vi "LEDs Streaming 2945 2955.vi"(0 "rx.parameters":T4={"rx.trigger select"=enum."Software", "rx.trigger enable"=FALSE, "rx.trigger sync enable"=FALSE, "rx.stream enable"=[FALSE, FALSE, FALSE, FALSE], "rx.software trigger"=FALSE, "rx.reset"=FALSE, "rx.abort"=FALSE, "rx.samples to acquire"=0, "rx.data sink"=enum."SFP Port 0", "rx.ddc parameters"=[{"output sample rate"=0.0, "delay"=0.0, "frequency shift"=0.0, "impairments"={"inline gain I"=0.0, "inline gain Q"=0.0, "cross gain I"=0.0, "cross gain Q"=0.0, "pre-gain offset I"=0.0, "pre-gain offset Q"=0.0, "post-gain offset I"=0.0, "post-gain offset Q"=0.0}, "phase"=0.0}, {"output sample rate"=0.0, "delay"=0.0, "frequency shift"=0.0, "impairments"={"inline gain I"=0.0, "inline gain Q"=0.0, "cross gain I"=0.0, "cross gain Q"=0.0, "pre-gain offset I"=0.0, "pre-gain offset Q"=0.0, "post-gain offset I"=0.0, "post-gain offset Q"=0.0}, "phase"=0.0}, {"output sample rate"=0.0, "delay"=0.0, "frequency shift"=0.0, "impairments"={"inline gain I"=0.0, "inline gain Q"=0.0, "cross gain I"=0.0, "cross gain Q"=0.0, "pre-gain offset I"=0.0, "pre-gain offset Q"=0.0, "post-gain offset I"=0.0, "post-gain offset Q"=0.0}, "phase"=0.0}, {"output sample rate"=0.0, "delay"=0.0, "frequency shift"=0.0, "impairments"={"inline gain I"=0.0, "inline gain Q"=0.0, "cross gain I"=0.0, "cross gain Q"=0.0, "pre-gain offset I"=0.0, "pre-gain offset Q"=0.0, "post-gain offset I"=0.0, "post-gain offset Q"=0.0}, "phase"=0.0}]} {"rx.ddc parameters"."frequency shift" format="%#.48g"}, 1 "rx.leds":T3, 5 "rx.status":T2={"rx.state"=enum."Idle", "rx.samples processed"=0, "rx.number of fifo overflows"=0, "rx.number of iq data overflows"=[0, 0, 0, 0], "rx.dsp reset done"=FALSE}) -> ()   [LabVIEW 2016]
uses:
  Stream Control State.ctl
  <vilib>/eio/EIONode/EIONode.xnode
  <vilib>/rvi/eio/common/nirviEmuTemplateMethod_errors.vi
  <instrlib>/_niInstr/Basic Elements/v1/FPGA/niInstr Basic Elements v1 FPGA.lvlib
  <instrlib>/_niInstr/Basic Elements/v1/FPGA/Private/Count Down U32.vi
  <instrlib>/_niInstr/DSP/v1/Shared/Public/IQ Impairments.ctl
  <instrlib>/_niInstr/DSP/v1/Shared/niInstr DSP v1 Shared.lvlib
  HOST/2954/SubVIs/Start Trigger.ctl
  DDC Parameters.ctl
  Rx Parameters.ctl
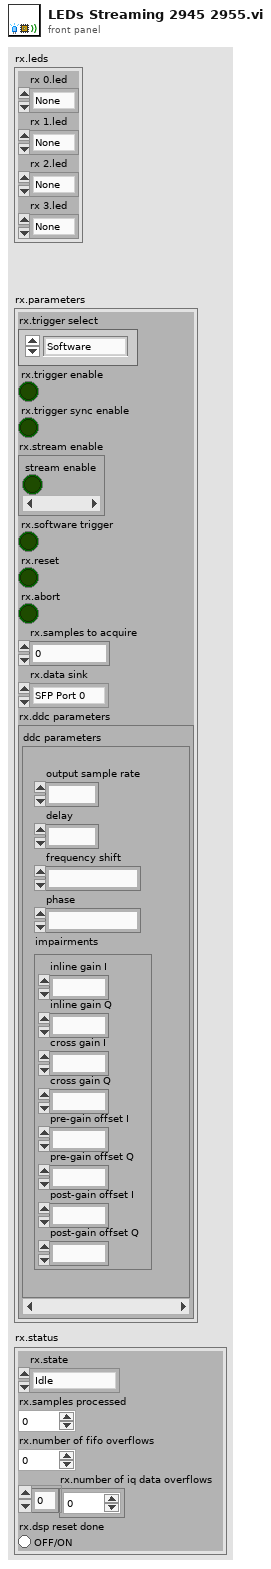
[diagram p1: front panel]
types:
  T1 = typedef "Stream Control State.ctl" = enum16{"Idle", "Active"}
  T2 = cluster{"rx.state":T1, "rx.samples processed":u32, "rx.number of fifo overflows":u32, "rx.number of iq data overflows":u64[], "rx.dsp reset done":bool}
  T3 = cluster{"rx 0.led":enum16{"None", "RF 0/RX 1", "RF 0/RX 2", "RF 1/RX 1", "RF 1/RX 2"}, "rx 1.led":enum16{"None", "RF 0/RX 1", "RF 0/RX 2", "RF 1/RX 1", "RF 1/RX 2"}, "rx 2.led":enum16{"None", "RF 0/RX 1", "RF 0/RX 2", "RF 1/RX 1", "RF 1/RX 2"}, "rx 3.led":enum16{"None", "RF 0/RX 1", "RF 0/RX 2", "RF 1/RX 1", "RF 1/RX 2"}}
  T4 = typedef "Rx Parameters.ctl" = cluster{"rx.trigger select":T5, "rx.trigger enable":bool, "rx.trigger sync enable":bool, "rx.stream enable":bool[], "rx.software trigger":bool, "rx.reset":bool, "rx.abort":bool, "rx.samples to acquire":u32, "rx.data sink":enum16{"SFP Port 0", "SFP Port 1", "Host"}, "rx.ddc parameters":T6[]}
  T5 = typedef "Start Trigger.ctl" = enum8{"Software", "Digital Edge", "Rx Start Trigger", "Tx Start Trigger", "Immediate", "Future Time Event"}
  T6 = typedef "DDC Parameters.ctl" = cluster{"output sample rate":fxp<+,48,1>, "delay":fxp<+/-,16,0>, "frequency shift":fxp<+/-,48,0>, "impairments":T7, "phase":fxp<+/-,21,0>}
  T7 = typedef "niInstr DSP v1 Shared.lvlib/IQ Impairments.ctl" = cluster{"inline gain I":fxp<+/-,18,1>, "inline gain Q":fxp<+/-,18,1>, "cross gain I":fxp<+/-,18,1>, "cross gain Q":fxp<+/-,18,1>, "pre-gain offset I":fxp<+/-,18,1>, "pre-gain offset Q":fxp<+/-,18,1>, "post-gain offset I":fxp<+/-,18,1>, "post-gain offset Q":fxp<+/-,18,1>}
  T8 = enum16{"None", "RF 0/RX 1", "RF 0/RX 2", "RF 1/RX 1", "RF 1/RX 2"}
  T9 = enum16{"None", "RF 0/RX 1", "RF 0/RX 2", "RF 1/RX 1", "RF 1/RX 2"}[]
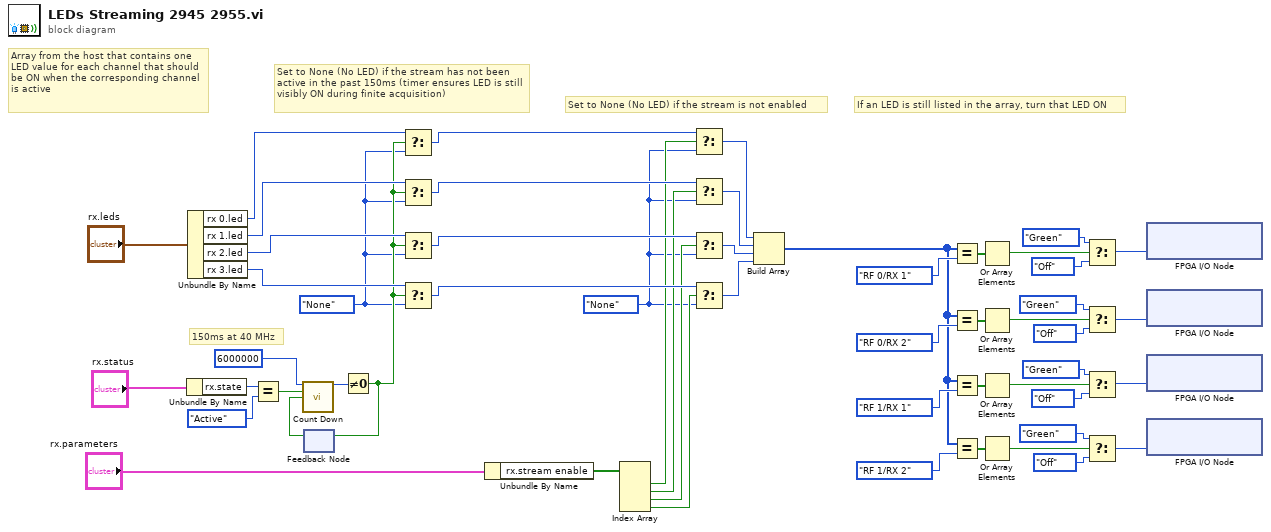
[diagram p0: block diagram]
diagram:
  w3 = T8."None" ("f")
  w10 = T8."None" ("f")
  # "If an LED is still listed in the array, turn that LED ON"
  # "Array from the host that contains one LED value for each channel that should be ON when the corresponding channel is active"
  # "Set to None (No LED) if the stream is not enabled"
  # "Set to None (No LED) if the stream has not been active in the past 150ms (timer ensures LED is still visibly ON during finite acquisition)"
  # "150ms at 40 MHz"
  n1 = Unbundle By Name("rx.status") -> ("rx.state"=w54:T1)
  n2 = Unbundle By Name("rx.leds") -> ("rx 0.led"=w12:T8, "rx 1.led"=w13:T8, "rx 2.led"=w14:T8, "rx 3.led"=w15:T8)
  n3 = Equal?(x=w54, y=Stream_Control_State."Active") -> (x = y?=w23:bool)
  n4 = feedback #1() -> (w20:bool)  [unwired: 1 in]
  n5 = call-poly <instrlib>:"Count Down.vi"("count in"=u32 6000000, "load"=w23, "decrement"=w20) -> ("count out"=w21:u32)  [unwired: 11 in, 1 out]
  n6 = Not Equal To 0?(x=w21) -> (x != 0?=w11:bool)
  n7 = feedback-in #1(w11) -> ()
  n8 = Select(t=w12, s=w11, f=w10) -> (s? t:f=w9:T8)
  n9 = Select(t=w13, s=w11, f=w10) -> (s? t:f=w8:T8)
  n10 = Select(t=w14, s=w11, f=w10) -> (s? t:f=w50:T8)
  n11 = Select(t=w15, s=w11, f=w10) -> (s? t:f=w49:T8)
  n12 = Unbundle By Name("rx.parameters") -> ("rx.stream enable"=w51:bool[])
  n13 = Index Array(array=w51) -> (element #1=w7:bool, element #2=w6:bool, element #3=w5:bool, element #4=w4:bool)  [unwired: 4 in]
  n14 = Select(t=w9, s=w7, f=w3) -> (s? t:f=w2:T8)
  n15 = Select(t=w8, s=w6, f=w3) -> (s? t:f=w1:T8)
  n16 = Select(t=w50, s=w5, f=w3) -> (s? t:f=w48:T8)
  n17 = Select(t=w49, s=w4, f=w3) -> (s? t:f=w47:T8)
  n18 = Build Array(w2, w1, w48, w47) -> (w31:T9)
  n19 = Equal?(x=w31, y=T8."RF 0/RX 1" ("f")) -> (x = y?=w45:bool[])
  n20 = Equal?(x=w31, y=T8."RF 0/RX 2" ("f")) -> (x = y?=w40:bool[])
  n21 = Equal?(x=w31, y=T8."RF 1/RX 1" ("f")) -> (x = y?=w37:bool[])
  n22 = Equal?(x=w31, y=T8."RF 1/RX 2" ("f")) -> (x = y?=w33:bool[])
  n23 = Or Array Elements(Boolean array=w45) -> (logical OR=w44:bool)
  n24 = Or Array Elements(Boolean array=w40) -> (logical OR=w41:bool)
  n25 = Or Array Elements(Boolean array=w37) -> (logical OR=w36:bool)
  n26 = Or Array Elements(Boolean array=w33) -> (logical OR=w25:bool)
  n27 = Select(t=enum8{"Off", "Green", "Red", "Amber"}."Green" ("LED/RF 0/TX1 RX1"), s=w44, f=enum8{"Off", "Green", "Red", "Amber"}."Off" ("LED/RF 0/TX1 RX1")) -> (s? t:f=w17:enum8{"Off", "Green", "Red", "Amber"})
  n28 = Select(t=enum8{"Off", "Green"}."Green" ("LED/RF 0/RX2"), s=w41, f=enum8{"Off", "Green"}."Off" ("LED/RF 0/RX2")) -> (s? t:f=w28:enum8{"Off", "Green"})
  n29 = Select(t=enum8{"Off", "Green", "Red", "Amber"}."Green" ("LED/RF 0/TX1 RX1"), s=w36, f=enum8{"Off", "Green", "Red", "Amber"}."Off" ("LED/RF 0/TX1 RX1")) -> (s? t:f=w16:enum8{"Off", "Green", "Red", "Amber"})
  n30 = Select(t=enum8{"Off", "Green"}."Green" ("LED/RF 0/RX2"), s=w25, f=enum8{"Off", "Green"}."Off" ("LED/RF 0/RX2")) -> (s? t:f=w24:enum8{"Off", "Green"})
  n31 = xnode "FPGA I/O Node"("LED/RF 0/RX1"=w17) -> ()  [unwired: 1 in, 1 out]
  n32 = xnode "FPGA I/O Node"("LED/RF 0/RX2"=w28) -> ()  [unwired: 1 in, 1 out]
  n33 = xnode "FPGA I/O Node"("LED/RF 1/RX1"=w16) -> ()  [unwired: 1 in, 1 out]
  n34 = xnode "FPGA I/O Node"("LED/RF 1/RX2"=w24) -> ()  [unwired: 1 in, 1 out]
